vi "sub_ekf_observation.vi"(9 "u":T1, 10 "xDR":T1, 11 "xTrue":T1) -> (0 "ud":T1, 1 "xDR":T1, 2 "z":T1, 3 "x_true out":T1)   [LabVIEW 2019]
uses:
  <vilib>/Analysis/Matrix/Datatypes/RealMatrix.ctl
  Ctrl/cmd_common.ctl
  <vilib>/Analysis/baseanly.llb/Real A x B.vi
  <vilib>/Analysis/Matrix/Numeric/Add/Add - RM,RM.vi
  <vilib>/Analysis/Matrix/NI_Matrix.lvlib
  <vilib>/ptbypt/NI_PtbyPt.lvlib
  <vilib>/Analysis/NI_AALBase.lvlib
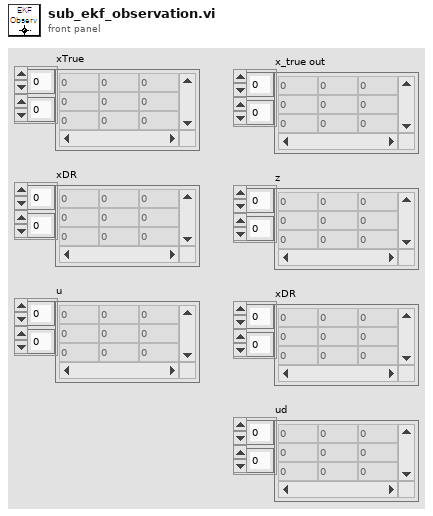
[diagram p1: front panel]
types:
  T1 = typedef "NI_Matrix.lvlib/RealMatrix.ctl" = dbl[][]
  T2 = typedef "cmd_common.ctl" = enum16{"read", "write"}
  T3 = cluster{"Q":T1, "R":T1, "input Noise":T1, "GPS noise":T1, "DT":dbl}
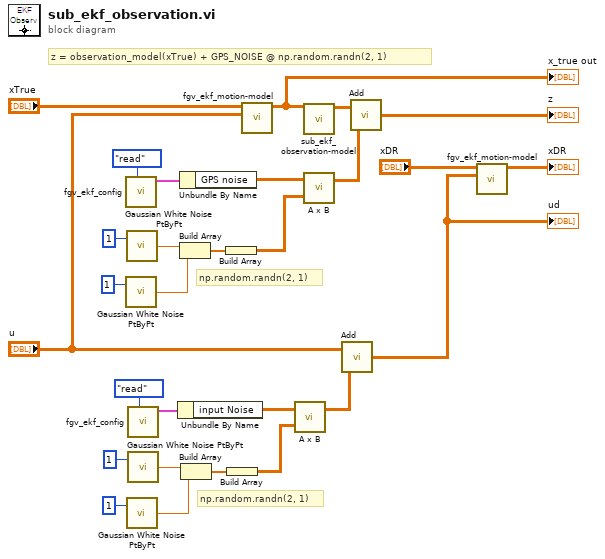
[diagram p0: block diagram]
diagram:
  # "np.random.randn(2, 1)"
  # "z = observation_model(xTrue) + GPS_NOISE @ np.random.randn(2, 1)"
  # "np.random.randn(2, 1)"
  n1 = call "fgv_ekf_config.vi"("cmd"=cmd_common."read") -> ("set var out"=w17:T3)  [unwired: 10 in]
  n2 = call <vilib>:"Gaussian White Noise PtByPt.vi"("standard deviation"=1 ("samples")) -> ("Gaussian white noise"=w21:dbl)  [unwired: 2 in]
  n3 = call <vilib>:"Gaussian White Noise PtByPt.vi"("standard deviation"=1 ("samples")) -> ("Gaussian white noise"=w22:dbl)  [unwired: 2 in]
  n4 = call <vilib>:"Gaussian White Noise PtByPt.vi"("standard deviation"=1 ("samples")) -> ("Gaussian white noise"=w10:dbl)  [unwired: 2 in]
  n5 = call "fgv_ekf_config.vi"("cmd"=cmd_common."read") -> ("set var out"=w5:T3)  [unwired: 10 in]
  n6 = call <vilib>:"Gaussian White Noise PtByPt.vi"("standard deviation"=1 ("samples")) -> ("Gaussian white noise"=w9:dbl)  [unwired: 2 in]
  n7 = Unbundle By Name(w5) -> ("input Noise"=w14:T1)
  n8 = Unbundle By Name(w17) -> ("GPS noise"=w18:T1)
  n9 = Build Array(w22, w21) -> (w23:dbl[])
  n10 = Build Array(w9, w10) -> (w8:dbl[])
  n11 = Build Array(w23) -> (w24:T1)
  n12 = Build Array(w8) -> (w13:T1)
  n13 = call "fgv_ekf_motion-model.vi"("u"="u", "x_true"="xTrue") -> ("x_true out"=w4:T1)  [unwired: 9 in]
  "x_true out" <- w4
  n14 = call-poly <vilib>:"A x B.vi"("B"=w13, "A"=w14) -> ("A x B"=w15:T1)  [unwired: 1 out]
  n15 = call "sub_ekf_observation-model.vi"("x_true"=w4) -> ("x_true out"=w25:T1)  [unwired: 10 in]
  n16 = call-poly <vilib>:"A x B.vi"("B"=w24, "A"=w18) -> ("A x B"=w26:T1)  [unwired: 1 out]
  n17 = call-poly <vilib>:"Add.vi"("Real Matrix B"=w15, "Real Matrix A"="u") -> ("A + B"=w2:T1)
  "ud" <- w2
  n18 = call-poly <vilib>:"Add.vi"("Real Matrix B"=w26, "Real Matrix A"=w25) -> ("A + B"=→"z":T1)
  n19 = call "fgv_ekf_motion-model.vi"("u"=w2, "x_true"="xDR") -> ("x_true out"=→"xDR":T1)  [unwired: 9 in]
